vi "Add Zenoh Error.vi"(8 "error in (no error)":errorcluster, 9 "String to Append":string, 10 "Error":T1, 11 "Insert Error":bool=TRUE) -> (0 "error out":errorcluster)   [LabVIEW 2021, in "Zenoh.lvclass"]
uses:
  Zenoh.lvclass
  typedef/Zenoh Errors.ctl
  Zenoh.lvclass/Zenoh.ctl
  <vilib>/CIF Foundation/CIF Utilities/Errors/Errors_CIF_U.lvlib
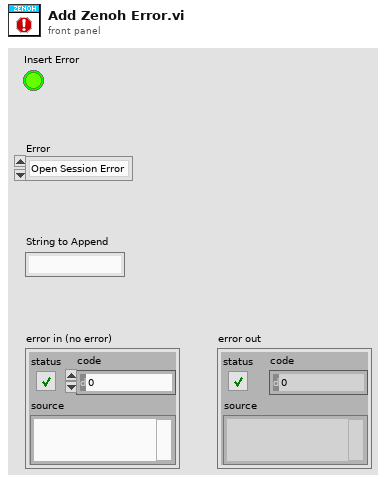
[diagram p1: front panel]
types:
  T1 = typedef "Zenoh.lvclass/Zenoh Errors.ctl" = enum16{"Open Session Error", "Open Subscription Error", "Declare Liveliness", "Query Keys", "File Error", "JSON Error", "Zenoh Runtime"}
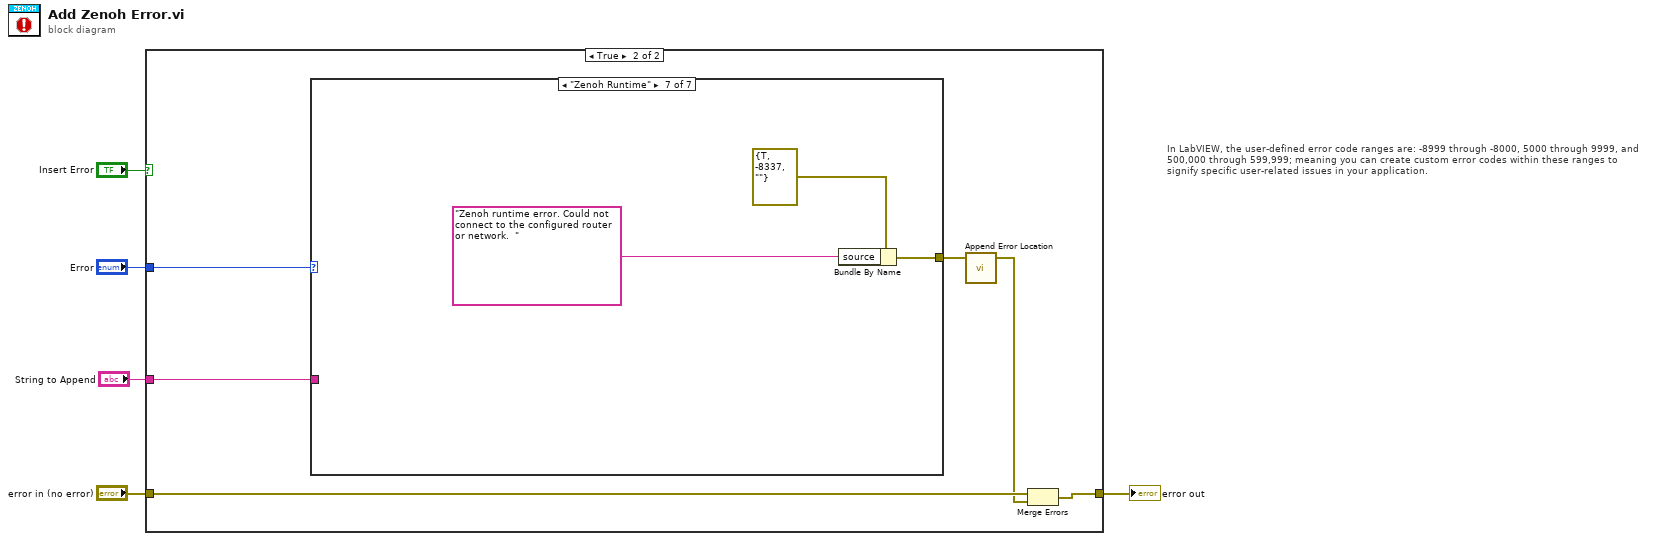
[diagram p0: block diagram]
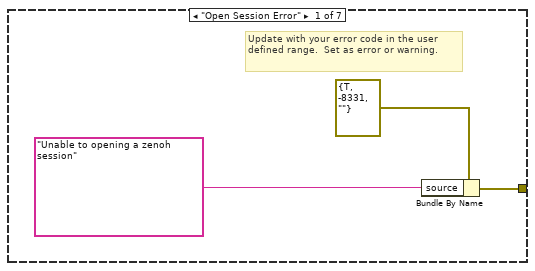
[diagram p3: hidden frame]
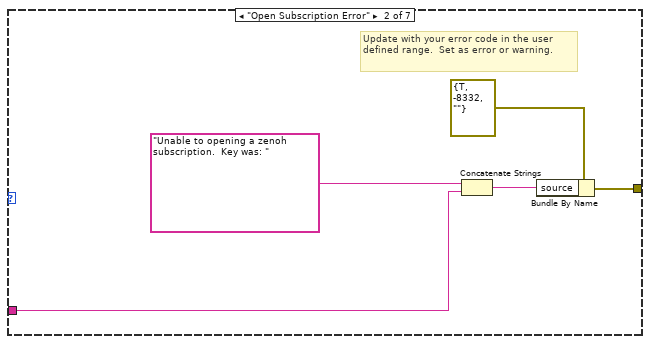
[diagram p4: hidden frame]
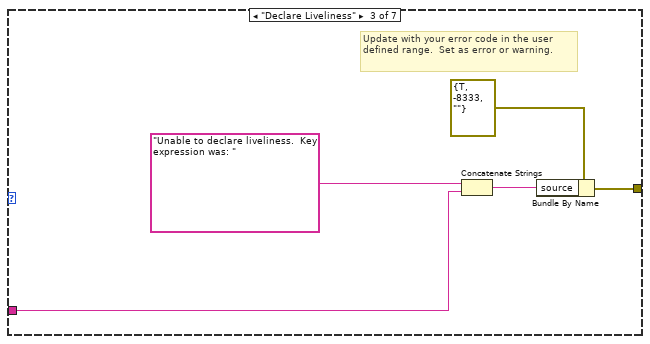
[diagram p5: hidden frame]
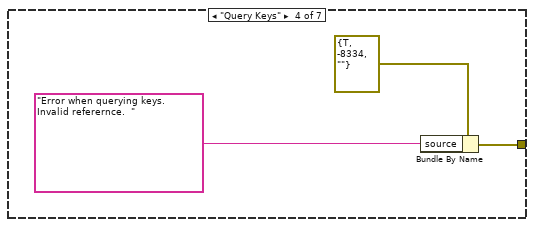
[diagram p6: hidden frame]
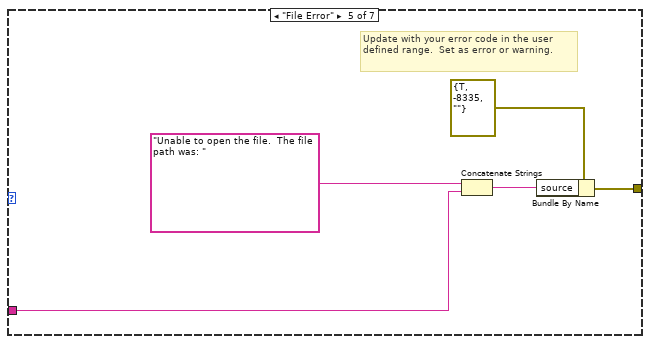
[diagram p7: hidden frame]
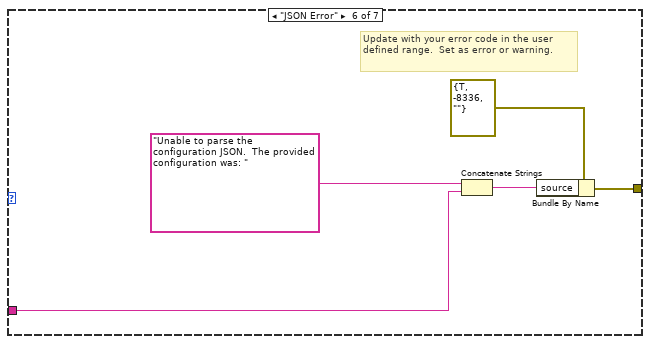
[diagram p8: hidden frame]
diagram:
  # "In LabVIEW, the user-defined error code ranges are: -8999 through -8000, 5000 through 9999, and 500,000 through 599,999; meaning you can create custom error codes within these ranges to signify specific user-related issues in your application."
  n1 = case shown="True" "Insert Error" {
    tunnel: [w6 w9] -> w4
    tunnel: "error in (no error)" -> [w6 w10]
    tunnel: "Error" -> [_ w12]
    tunnel: "String to Append" -> [_ w11]
    frame False {
    }
    frame True {
      n2 = case shown="\"Zenoh Runtime\"" w12 {
        tunnel: w11 -> [_ w16 w21 _ w29 w34 _]
        tunnel: [w14 w19 w24 w27 w32 w37 w40] -> w8
        frame "Open Session Error" {
          # "Update with your error code in the user defined range.  Set as error or warning."
          n3 = Bundle By Name(cluster=errorcluster {"status"=TRUE, "code"=-8331, "source"=""} ("Invalid ID"), "source"="Unable to opening a zenoh session") -> (w14:errorcluster)
        }
        frame "Open Subscription Error" {
          # "Update with your error code in the user defined range.  Set as error or warning."
          n4 = Concatenate Strings("Unable to opening a zenoh subscription.  Key was: " ("source"), w16) -> (w17:string)
          n5 = Bundle By Name(cluster=errorcluster {"status"=TRUE, "code"=-8332, "source"=""} ("Invalid ID"), "source"=w17) -> (w19:errorcluster)
        }
        frame "Declare Liveliness" {
          # "Update with your error code in the user defined range.  Set as error or warning."
          n6 = Concatenate Strings("Unable to declare liveliness.  Key expression was: " ("source"), w21) -> (w22:string)
          n7 = Bundle By Name(cluster=errorcluster {"status"=TRUE, "code"=-8333, "source"=""} ("Invalid ID"), "source"=w22) -> (w24:errorcluster)
        }
        frame "Query Keys" {
          n8 = Bundle By Name(cluster=errorcluster {"status"=TRUE, "code"=-8334, "source"=""} ("Invalid ID"), "source"="Error when querying keys.  Invalid referernce.  ") -> (w27:errorcluster)
        }
        frame "File Error" {
          # "Update with your error code in the user defined range.  Set as error or warning."
          n9 = Concatenate Strings("Unable to open the file.  The file path was: " ("source"), w29) -> (w30:string)
          n10 = Bundle By Name(cluster=errorcluster {"status"=TRUE, "code"=-8335, "source"=""} ("Invalid ID"), "source"=w30) -> (w32:errorcluster)
        }
        frame "JSON Error" {
          # "Update with your error code in the user defined range.  Set as error or warning."
          n11 = Concatenate Strings("Unable to parse the configuration JSON.  The provided configuration was: " ("source"), w34) -> (w35:string)
          n12 = Bundle By Name(cluster=errorcluster {"status"=TRUE, "code"=-8336, "source"=""} ("Invalid ID"), "source"=w35) -> (w37:errorcluster)
        }
        frame "Zenoh Runtime" {
          n13 = Bundle By Name(cluster=errorcluster {"status"=TRUE, "code"=-8337, "source"=""} ("Invalid ID"), "source"="Zenoh runtime error. Could not connect to the configured router or network.  ") -> (w40:errorcluster)
        }
      }
      n14 = call <vilib>:"Append Error Location.vi"("error in (no error)"=w8) -> ("error out"=w7:errorcluster)  [unwired: 4 in]
      n15 = Merge Errors(w10, w7) -> (w9:errorcluster)
    }
  }
  "error out" <- w4
